vi "Process coin.vi"(8 "error in (no error)":errorcluster, 10 "Monedas":cluster{"1":bool, "2":bool, "5":bool}, 11 "MXN actor in":refnum<class "MXN actor.lvclass">) -> (0 "error out":errorcluster, 3 "MXN actor out":refnum<class "MXN actor.lvclass">)   [LabVIEW 2020, in "MXN actor.lvlib" / "MXN actor.lvclass"]
uses:
  MXN actor.lvclass
  C:/Program Files/National Instruments/LabVIEW 2020/vi.lib/ActorFramework/Actor/Actor.lvclass
  <vilib>/ActorFramework/Actor/Actor.lvclass/Actor.ctl
  MXN actor.lvclass/MXN actor.ctl
  UI Actor Messages/credit update Msg/credit update Msg.lvclass/credit update Msg.ctl
  <vilib>/ActorFramework/Message Enqueuer/Message Enqueuer.lvclass/Message Enqueuer.ctl
  <vilib>/ActorFramework/Message Enqueuer/Enqueue.vi
  UI Actor Messages/credit update Msg/credit update Msg.lvclass
  C:/Program Files/National Instruments/LabVIEW 2020/vi.lib/ActorFramework/Message/Message.lvclass
  <vilib>/ActorFramework/Message Priority Queue/Priority Enqueue.vi
  <vilib>/ActorFramework/Actor/Actor.lvclass
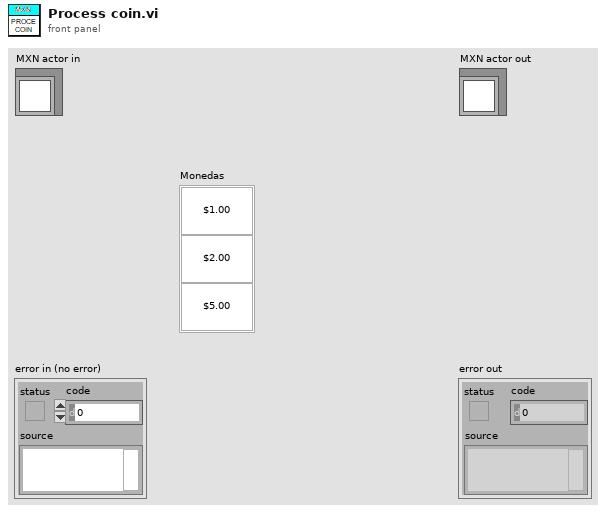
[diagram p1: front panel]
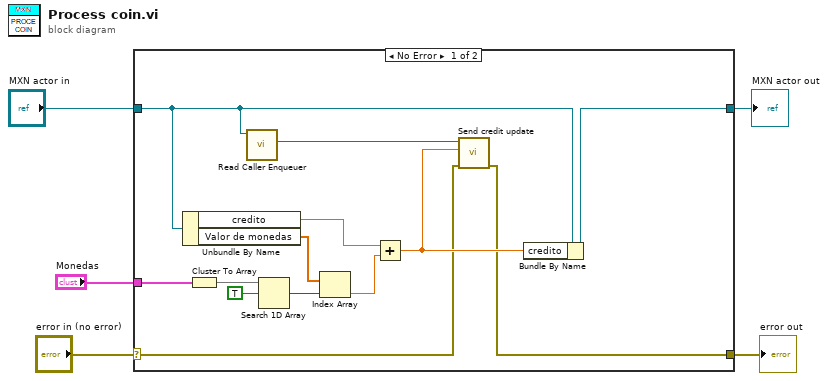
[diagram p0: block diagram]
diagram:
  n1 = case shown="No Error" "error in (no error)" {
    selector: "error in (no error)" -> [w7 w20]
    tunnel: [w6 w20] -> w4
    tunnel: [w11 w19] -> w2
    tunnel: "MXN actor in" -> [w10 w19]
    tunnel: "Monedas" -> [w18 _]
    frame No Error {
      n2 = Unbundle By Name(w10) -> ("credito"=w13:dbl, "Valor de monedas"=w15:dbl[])
      n3 = Cluster To Array(cluster=w18) -> (array=w17:bool[])
      n4 = call <vilib>:"Read Caller Enqueuer.vi"("Actor"=w10) -> ("Caller Enqueuer"=w9:refnum<class "Message Enqueuer.lvclass">)  [unwired: 10 in]
      n5 = Search 1D Array(1D array=w17, element=TRUE) -> (index of element=w14:i32)  [unwired: 1 in]
      n6 = Index Array(array=w15, index=w14) -> (element=w12:dbl)
      n7 = Add(x=w13, y=w12) -> (x+y=w8:dbl)
      n8 = call "Send credit update.vi"("error in (no error)"=w7, "credito"=w8, "Message Enqueuer"=w9) -> ("error out"=w6:errorcluster)  [unwired: 7 in, 1 out]
      n9 = Bundle By Name(cluster=w10, "credito"=w8) -> (w11:refnum<class "MXN actor.lvclass">)
    }
    frame Error {
    }
  }
  "error out" <- w4
  "MXN actor out" <- w2
